vi "Has Trailing Slash.vi"(4 "Path String in":string) -> (6 "Has Trailing Slash":bool, 7 "Path String":string)   [LabVIEW 2020, in "URI.lvlib"]
uses:
  URI.lvlib
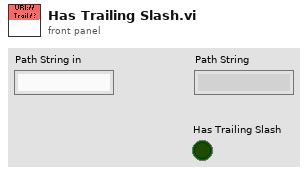
[diagram p1: front panel]
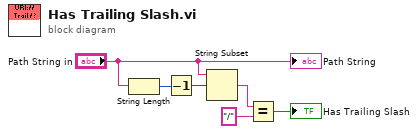
[diagram p0: block diagram]
diagram:
  n1 = String Length(string="Path String in") -> (length=w6:i32)
  n2 = Decrement(x=w6) -> (x-1=w5:i32)
  n3 = String Subset(string="Path String in", offset (0)=w5) -> (substring=w3:string)  [unwired: 1 in]
  n4 = Equal?(x=w3, y="/") -> (x = y?=→"Has Trailing Slash":bool)
  "Path String" <- "Path String in"
